vi "MeasureSource.vi"(8 "error in (no error)":errorcluster, 10 "Enable?":bool=TRUE, 11 "Input parameters":T1={"Measurement type"=enum."Test", "Sensor type"=enum."HPK_8in_256", "Identifier"="test.txt", "Open after execution?"=FALSE, "Plot after execution?"=FALSE, "Display channel"=0, "Voltage Delay (s)"=0.5, "Switch Delay (s)"=0.01, "VISA resource name source"="", "VISA resource name DMM"="", "VISA resource name LCR"="", "Compliance  Level (uA)"=10.0, "Voltage Limit (V)"=1000.0, "Data storage location"="", "Scan voltages"="", "Use source as DMM?"=FALSE, "Single channel?"=FALSE, "LCR signal frequenzy (Hz)"=10.0, "DMM device"=enum."Keithley2001"} {"Voltage Limit (V)" format="%#_13g"; "Voltage Delay (s)" format="%#_13g"; "Switch Delay (s)" format="%#_13g"}) -> (0 "error out":errorcluster, 3 "Total current":dbl, 5 "Actual voltage":dbl)   [LabVIEW 2016]
uses:
  Input_parameters.ctl
  <instrlib>/Keithley 24XX/Public/Data/Read (Single Point).vi
  <instrlib>/Keithley 24XX/Keithley 24XX.lvlib
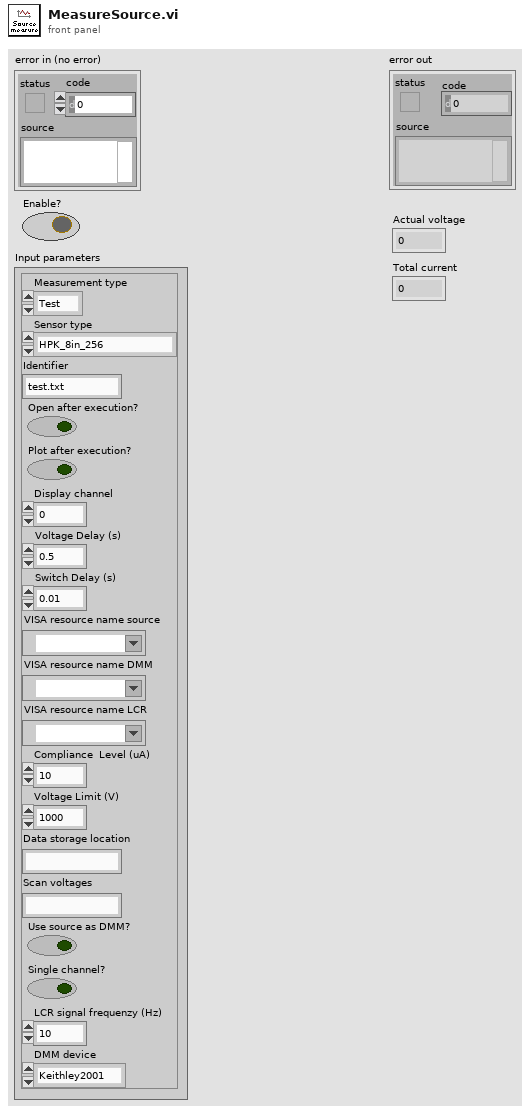
[diagram p1: front panel]
types:
  T1 = typedef "Input_parameters.ctl" = cluster{"Measurement type":enum16{"IV", "CV", "Test"}, "Sensor type":enum16{"HPK_6in_135", "HPK_8in_256", "INF_8in_256", "Diode"}, "Identifier":string, "Open after execution?":bool, "Plot after execution?":bool, "Display channel":i32, "Voltage Delay (s)":dbl, "Switch Delay (s)":dbl, "VISA resource name source":refnum<visa-resource-name>, "VISA resource name DMM":refnum<visa-resource-name>, "VISA resource name LCR":refnum<visa-resource-name>, "Compliance  Level (uA)":dbl, "Voltage Limit (V)":dbl, "Data storage location":string, "Scan voltages":string, "Use source as DMM?":bool, "Single channel?":bool, "LCR signal frequenzy (Hz)":dbl, "DMM device":enum16{"Keithley2001", "Keithley2450", "Keithley2410"}}
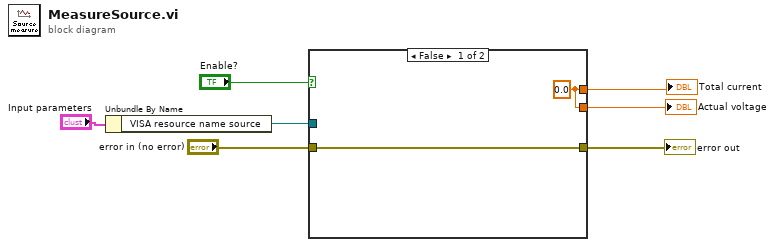
[diagram p0: block diagram]
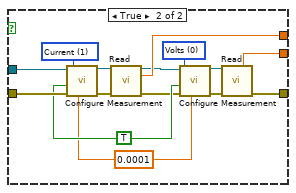
[diagram p2: hidden frame]
diagram:
  n1 = Unbundle By Name("Input parameters") -> ("VISA resource name source"=w3:refnum<visa-resource-name>)
  n2 = case shown="False" "Enable?" {
    tunnel: [w9 w24] -> w7
    tunnel: [w9 w23] -> w5
    tunnel: [w8 w22] -> w4
    tunnel: w3 -> [_ w21]
    tunnel: "error in (no error)" -> [w8 w20]
    frame False {
      w9 = sgl 0.0 ("Current")
    }
    frame True {
      w11 = u16 0 items=["Volts", "Current", "Resistance"] ("Function (0: Volts)")
      w19 = u16 1 items=["Volts", "Current", "Resistance"] ("Function (0: Volts)")
      w16 = TRUE ("Enable Auto Range (T:Enable)")
      w10 = 0.0001 ("Manual Range (1.0)")
      n3 = call <instrlib>:"Configure Measurement.vi"("Manual Range (1.0)"=w10, "error in (no error)"=w20, "Enable Auto Range (T:Enable)"=w16, "Function (0: Volts)"=w19, "VISA resource name"=w21) -> ("error out"=w17:errorcluster, "VISA resource name out"=w18:refnum<visa-resource-name>)  [unwired: 5 in]
      n4 = call-poly <instrlib>:"Read.vi"("VISA resource name"=w18, "error in (no error)"=w17) -> ("VISA resource name out"=w12:refnum<visa-resource-name>, "Current"=w24:sgl, "error out"=w15:errorcluster)  [unwired: 7 in, 4 out]
      n5 = call <instrlib>:"Configure Measurement.vi"("Manual Range (1.0)"=w10, "error in (no error)"=w15, "Enable Auto Range (T:Enable)"=w16, "Function (0: Volts)"=w11, "VISA resource name"=w12) -> ("error out"=w14:errorcluster, "VISA resource name out"=w13:refnum<visa-resource-name>)  [unwired: 5 in]
      n6 = call-poly <instrlib>:"Read.vi"("VISA resource name"=w13, "error in (no error)"=w14) -> ("Voltage"=w23:sgl, "error out"=w22:errorcluster)  [unwired: 7 in, 5 out]
    }
  }
  "Total current" <- w7
  "Actual voltage" <- w5
  "error out" <- w4
